vi "LVPortControlBindingGlobals.vi"() -> ()   [LabVIEW 2017]
panel:
  out "PropertyUpdatingByID":variant
  out "PropertyBindingByID":variant
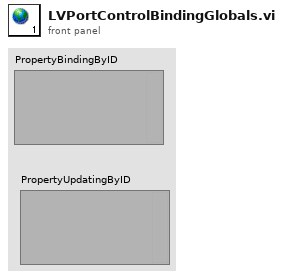
[diagram p1: front panel]
diagram:
